vi "generate_checksum.vi"(10 "message":string) -> (2 "checksum":string)   [LabVIEW 2018]
doc: "Generate the checksum sent with the command packet for validation."
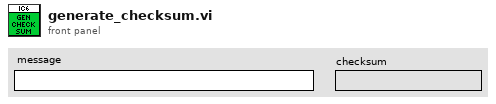
[diagram p1: front panel]
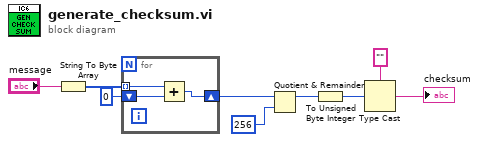
[diagram p0: block diagram]
diagram:
  n1 = String To Byte Array(string="message") -> (unsigned byte array=w5:u8[])
  n2 = for {
    tunnel: w5 -> [w12] mode=indexing
    shift-right: [w10] -> w3
    shift-left: u32 0 -> [w11]
    n3 = Add(x=w12, y=w11) -> (x+y=w10:u32)
  }
  n4 = Quotient & Remainder(x=w3, y=u32 256) -> (x-y*floor(x/y)=w1:u32)  [unwired: 1 out]
  n5 = To Unsigned Byte Integer(number=w1) -> (unsigned 8bit integer=w2:u8)
  n6 = Type Cast(type="", x=w2) -> (*(type *) &x=→"checksum":string)
